vi "Caculate Tray Point.vi"() -> ()   [LabVIEW 2019]
uses:
  global/Tray_ArrAndData.vi
panel:
  out "TrayAreaPt":T1(array[cluster])
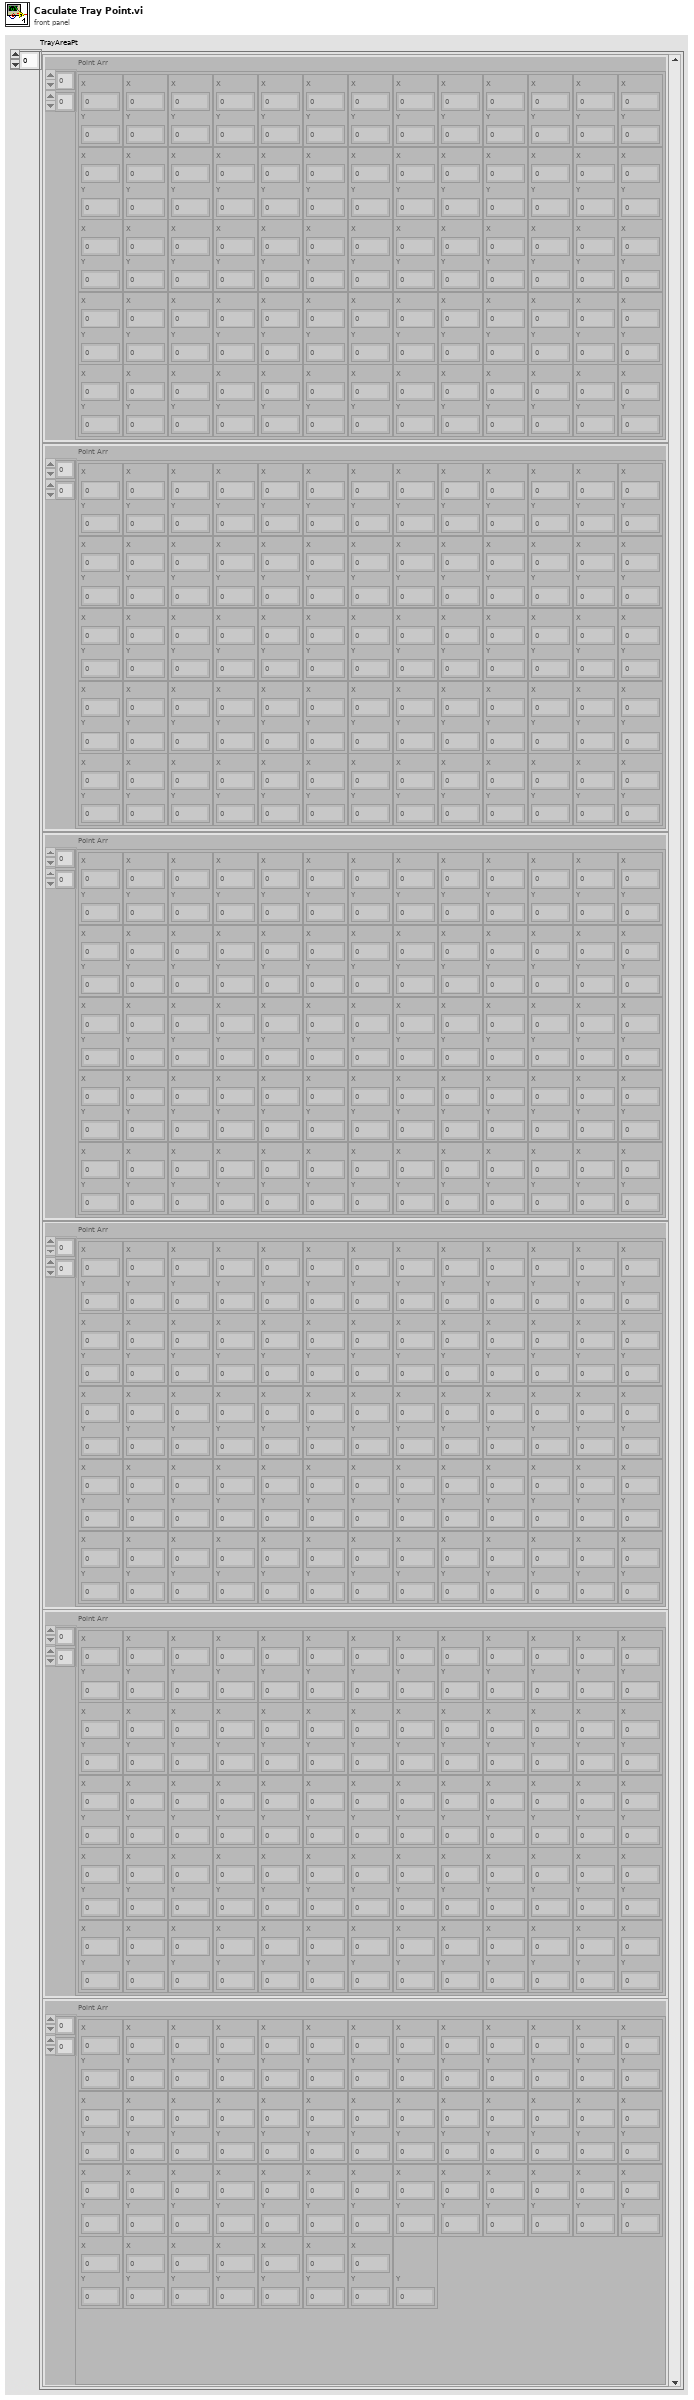
[diagram p1: front panel]
types:
  T1 = cluster{" Point Arr":cluster{"X":sgl, "Y":sgl}[][]}[]
  T2 = enum16{"Initial", "Load", "Save", "Read", "WriteSpeed", "WritePoint"}
  T3 = cluster{"Laser Point 2D Arr":cluster{"X":sgl, "Y":sgl}[][]}
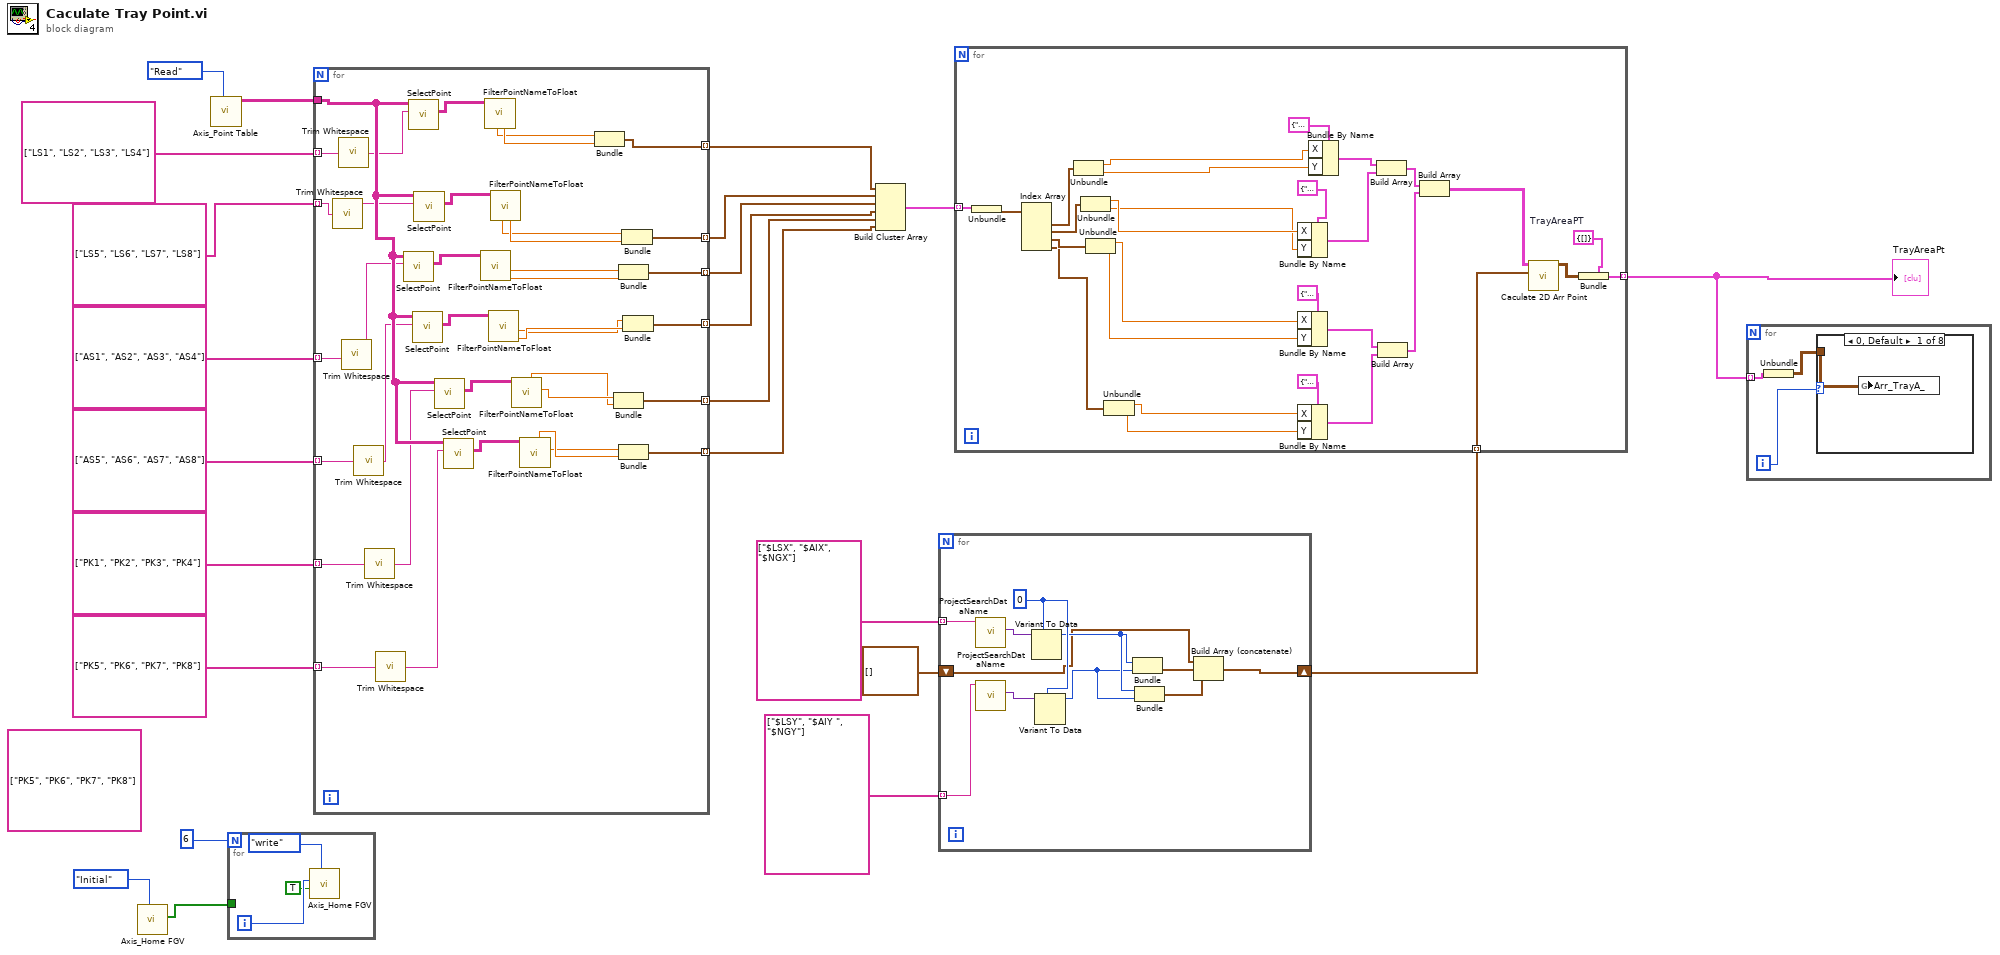
[diagram p0: block diagram]
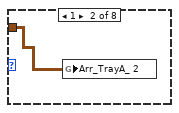
[diagram p2: hidden frame]
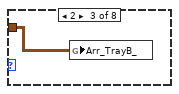
[diagram p3: hidden frame]
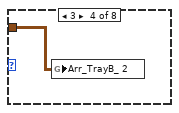
[diagram p4: hidden frame]
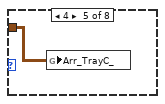
[diagram p5: hidden frame]
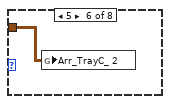
[diagram p6: hidden frame]
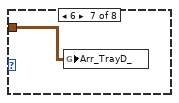
[diagram p7: hidden frame]
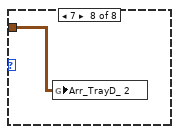
[diagram p8: hidden frame]
diagram:
  (unwired) string[] ["PK5", "PK6", "PK7", "PK8"]
  n1 = call "Axis_Home FGV.vi"("Enum"=enum16{"Initial", "write", "read"}."Initial") -> ("HMSStatus"=w5:bool[])  [unwired: 9 in, 1 out]
  n2 = call "Axis_Point Table.vi"("Enum"=T2."Read") -> ("RobotPoint"=w22:string[][])  [unwired: 8 in, 2 out]
  n3 = for {
    N: 6 -> [_]
    tunnel: w5 -> [_]
    i -> [w25]
    n4 = call "Axis_Home FGV.vi"("Enum"=enum16{"Initial", "write", "read"}."write", "Home"=TRUE, "Axis"=w25) -> ()  [unwired: 7 in, 2 out]
  }
  n5 = for {
    tunnel: w22 -> [w57]
    tunnel: string[] ["LS1", "LS2", "LS3", "LS4"] -> [w63] mode=indexing
    tunnel: string[] ["LS5", "LS6", "LS7", "LS8"] -> [w62] mode=indexing
    tunnel: string[] ["AS1", "AS2", "AS3", "AS4"] -> [w61] mode=indexing
    tunnel: string[] ["AS5", "AS6", "AS7", "AS8"] -> [w60] mode=indexing
    tunnel: string[] ["PK1", "PK2", "PK3", "PK4"] -> [w59] mode=indexing
    tunnel: string[] ["PK5", "PK6", "PK7", "PK8"] -> [w58] mode=indexing
    tunnel: [w52] -> w15 mode=indexing
    tunnel: [w51] -> w14 mode=indexing
    tunnel: [w50] -> w13 mode=indexing
    tunnel: [w49] -> w12 mode=indexing
    tunnel: [w48] -> w11 mode=indexing
    tunnel: [w47] -> w10 mode=indexing
    n6 = call <vilib>:"Trim Whitespace.vi"("string"=w62) -> ("trimmed string"=w39:string)  [unwired: 1 in]
    n7 = call <vilib>:"Trim Whitespace.vi"("string"=w63) -> ("trimmed string"=w46:string)  [unwired: 1 in]
    n8 = call <vilib>:"Trim Whitespace.vi"("string"=w61) -> ("trimmed string"=w38:string)  [unwired: 1 in]
    n9 = call <vilib>:"Trim Whitespace.vi"("string"=w60) -> ("trimmed string"=w37:string)  [unwired: 1 in]
    n10 = call <vilib>:"Trim Whitespace.vi"("string"=w59) -> ("trimmed string"=w36:string)  [unwired: 1 in]
    n11 = call <vilib>:"Trim Whitespace.vi"("string"=w58) -> ("trimmed string"=w35:string)  [unwired: 1 in]
    n12 = call "SelectPoint.vi"("PointName"=w38, "RobotPointsTableIn"=w57) -> ("RobotPointsOut"=w43:string[][])  [unwired: 7 in, 2 out]
    n13 = call "SelectPoint.vi"("PointName"=w46, "RobotPointsTableIn"=w57) -> ("RobotPointsOut"=w45:string[][])  [unwired: 7 in, 2 out]
    n14 = call "SelectPoint.vi"("PointName"=w37, "RobotPointsTableIn"=w57) -> ("RobotPointsOut"=w42:string[][])  [unwired: 7 in, 2 out]
    n15 = call "SelectPoint.vi"("PointName"=w39, "RobotPointsTableIn"=w57) -> ("RobotPointsOut"=w44:string[][])  [unwired: 7 in, 2 out]
    n16 = call "SelectPoint.vi"("PointName"=w36, "RobotPointsTableIn"=w57) -> ("RobotPointsOut"=w41:string[][])  [unwired: 7 in, 2 out]
    n17 = call "SelectPoint.vi"("PointName"=w35, "RobotPointsTableIn"=w57) -> ("RobotPointsOut"=w40:string[][])  [unwired: 7 in, 2 out]
    n18 = call "FilterPointNameToFloat.vi"("RobotPoints in"=w43) -> ("U"=w33:dbl, "Z"=w34:dbl)  [unwired: 4 in, 5 out]
    n19 = call "FilterPointNameToFloat.vi"("RobotPoints in"=w45) -> ("Y"=w56:dbl, "X"=w55:dbl)  [unwired: 4 in, 5 out]
    n20 = call "FilterPointNameToFloat.vi"("RobotPoints in"=w42) -> ("U"=w32:dbl, "Z"=w31:dbl)  [unwired: 4 in, 5 out]
    n21 = call "FilterPointNameToFloat.vi"("RobotPoints in"=w44) -> ("Y"=w54:dbl, "X"=w53:dbl)  [unwired: 4 in, 5 out]
    n22 = call "FilterPointNameToFloat.vi"("RobotPoints in"=w41) -> ("V"=w29:dbl, "W"=w28:dbl)  [unwired: 4 in, 5 out]
    n23 = call "FilterPointNameToFloat.vi"("RobotPoints in"=w40) -> ("V"=w27:dbl, "W"=w30:dbl)  [unwired: 4 in, 5 out]
    n24 = Bundle("X"=w55, "Y"=w56) -> (w52:cluster{"X":dbl, "Y":dbl})  [unwired: 1 in]
    n25 = Bundle("V"=w29, "W"=w28) -> (w48:cluster{"V":dbl, "W":dbl})  [unwired: 1 in]
    n26 = Bundle("Z"=w34, "U"=w33) -> (w50:cluster{"Z":dbl, "U":dbl})  [unwired: 1 in]
    n27 = Bundle("V"=w27, "W"=w30) -> (w47:cluster{"V":dbl, "W":dbl})  [unwired: 1 in]
    n28 = Bundle("X"=w53, "Y"=w54) -> (w51:cluster{"X":dbl, "Y":dbl})  [unwired: 1 in]
    n29 = Bundle("Z"=w31, "U"=w32) -> (w49:cluster{"Z":dbl, "U":dbl})  [unwired: 1 in]
  }
  n30 = Build Cluster Array(w15, w14, w13, w12, w11, w10) -> (w9:cluster{cluster{"V":dbl, "W":dbl}[]}[])
  n31 = for {
    tunnel: string[] ["$LSX", "$AIX", "$NGX"] -> [w74] mode=indexing
    tunnel: string[] ["$LSY", "$AIY ", "$NGY"] -> [w73] mode=indexing
    shift-right: [w65] -> w8
    shift-left: cluster{i32, i32}[] [] -> [w64]
    w70 = 0
    n32 = call "ProjectSearchDataName.vi"("element"=w74) -> ("variant"=w72:variant)  [unwired: 8 in, 2 out]
    n33 = call "ProjectSearchDataName.vi"("element"=w73) -> ("variant"=w71:variant)  [unwired: 8 in, 2 out]
    n34 = Variant To Data(type=w70, Variant=w72) -> (data=w69:i32)  [unwired: 1 in, 1 out]
    n35 = Variant To Data(type=w70, Variant=w71) -> (data=w68:i32)  [unwired: 1 in, 1 out]
    n36 = Bundle(w69, w68) -> (w67:cluster{i32, i32})  [unwired: 1 in]
    n37 = Bundle(w69, w68) -> (w66:cluster{i32, i32})  [unwired: 1 in]
    n38 = Build Array (concatenate)(w64, w67, w66) -> (w65:cluster{i32, i32}[])
  }
  n39 = for {
    tunnel: w9 -> [w103] mode=indexing
    tunnel: w8 -> [w78] mode=indexing
    tunnel: [w75] -> w4 mode=indexing
    w76 = T3 {"Laser Point 2D Arr"=[]}  # TrayAreaPT
    n40 = Unbundle(w103) -> (w102:cluster{"V":dbl, "W":dbl}[])
    n41 = Index Array(array=w102) -> (element #1=w101:cluster{"V":dbl, "W":dbl}, element #2=w98:cluster{"V":dbl, "W":dbl}, element #3=w100:cluster{"V":dbl, "W":dbl}, element #4=w99:cluster{"V":dbl, "W":dbl})  [unwired: 4 in]
    n42 = Unbundle(w101) -> ("V"=w93:dbl, "W"=w92:dbl)
    n43 = Unbundle(w98) -> ("V"=w91:dbl, "W"=w90:dbl)
    n44 = Unbundle(w100) -> ("V"=w89:dbl, "W"=w88:dbl)
    n45 = Unbundle(w99) -> ("V"=w87:dbl, "W"=w86:dbl)
    n46 = Bundle By Name(cluster=cluster{"Name":string, "X":dbl, "Y":dbl} {"Name"="POINT 2", "X"=0.0, "Y"=0.0} ("LaserPoint"), "X"=w91, "Y"=w90) -> (w84:cluster{"Name":string, "X":dbl, "Y":dbl})
    n47 = Bundle By Name(cluster=cluster{"Name":string, "X":dbl, "Y":dbl} {"Name"="POINT 3", "X"=0.0, "Y"=0.0} ("LaserPoint"), "X"=w89, "Y"=w88) -> (w83:cluster{"Name":string, "X":dbl, "Y":dbl})
    n48 = Bundle By Name(cluster=cluster{"Name":string, "X":dbl, "Y":dbl} {"Name"="POINT 4", "X"=0.0, "Y"=0.0} ("LaserPoint"), "X"=w87, "Y"=w86) -> (w82:cluster{"Name":string, "X":dbl, "Y":dbl})
    n49 = Bundle By Name(cluster=cluster{"Name":string, "X":dbl, "Y":dbl} {"Name"="POINT 1", "X"=0.0, "Y"=0.0} ("LaserPoint"), "X"=w93, "Y"=w92) -> (w85:cluster{"Name":string, "X":dbl, "Y":dbl})
    n50 = Build Array(w85, w84) -> (w81:cluster{"Name":string, "X":dbl, "Y":dbl}[])
    n51 = Build Array(w83, w82) -> (w80:cluster{"Name":string, "X":dbl, "Y":dbl}[])
    n52 = Build Array(w81, w80) -> (w79:cluster{"Name":string, "X":dbl, "Y":dbl}[][])
    n53 = call "Caculate 2D Arr Point.vi"("Array"=w78, "Set Laser Point Arr"=w79) -> ("Laser Point 2D Arr"=w77:cluster{"X":sgl, "Y":sgl}[][])  [unwired: 9 in]
    n54 = Bundle(cluster=w76, "Laser Point 2D Arr"=w77) -> (w75:T3)
  }
  "TrayAreaPt" <- w4
  n55 = for {
    tunnel: w4 -> [w106] mode=indexing
    i -> [w104]
    n56 = Unbundle(w106) -> ("Laser Point 2D Arr"=w105:cluster{"X":sgl, "Y":sgl}[][])
    n57 = case shown="0, Default" w104 {
      tunnel: w105 -> [w107 w108 w109 w110 w111 w112 w113 w114]
      frame 0, Default {
        n58 = global write "Tray_ArrAndData.vi" "Arr_TrayA_"(w107) -> ()
      }
      frame 1 {
        n59 = global write "Tray_ArrAndData.vi" "Arr_TrayA_ 2"(w108) -> ()
      }
      frame 2 {
        n60 = global write "Tray_ArrAndData.vi" "Arr_TrayB_"(w109) -> ()
      }
      frame 3 {
        n61 = global write "Tray_ArrAndData.vi" "Arr_TrayB_ 2"(w110) -> ()
      }
      frame 4 {
        n62 = global write "Tray_ArrAndData.vi" "Arr_TrayC_"(w111) -> ()
      }
      frame 5 {
        n63 = global write "Tray_ArrAndData.vi" "Arr_TrayC_ 2"(w112) -> ()
      }
      frame 6 {
        n64 = global write "Tray_ArrAndData.vi" "Arr_TrayD_"(w113) -> ()
      }
      frame 7 {
        n65 = global write "Tray_ArrAndData.vi" "Arr_TrayD_ 2"(w114) -> ()
      }
    }
  }
